vi "CreateLogStopNode.vi"(7 "DOM Document":refnum<k20>, 8 "Error In":errorcluster, 11 "Log Stop Configuration":T1={"Trigger Type"=enum."User", "Timer (sec)"=0.0, "File Size (MB)"=256, "Digital IO Line"=1, "Digital IO Edge"=enum."Rising"}) -> (0 "Error Out":errorcluster, 3 "Stop Node":refnum<k20>)   [LabVIEW 2013]
uses:
  LogStopConfiguration.ctl
  LogStopTriggerType.ctl
  LogDigitalIOTriggerEdge.ctl
  libs/LV-Utilities/LV-Utilities.lvlib
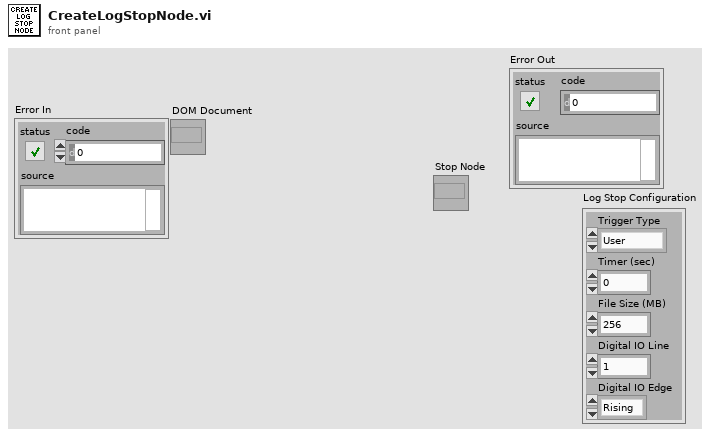
[diagram p1: front panel]
types:
  T1 = typedef "LogStopConfiguration.ctl" = cluster{"Trigger Type":T2, "Timer (sec)":dbl, "File Size (MB)":u32, "Digital IO Line":u8, "Digital IO Edge":T3}
  T2 = typedef "LogStopTriggerType.ctl" = enum16{"None", "User", "Timer", "File Size", "Digital IO"}
  T3 = typedef "LogDigitalIOTriggerEdge.ctl" = enum16{"Rising", "Falling"}
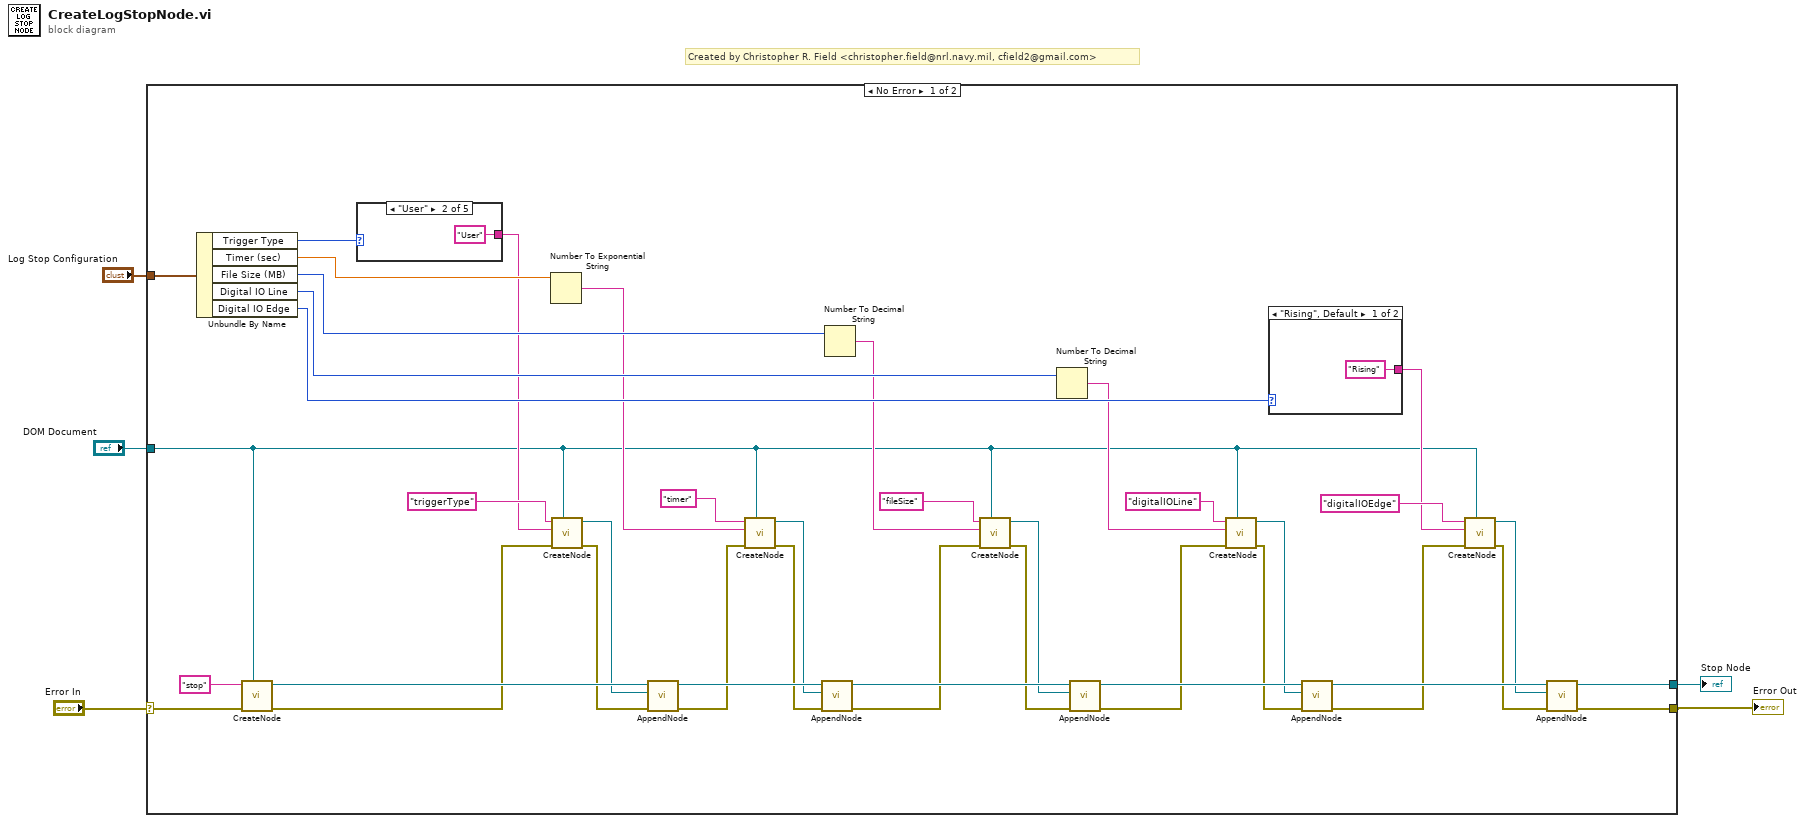
[diagram p0: block diagram]
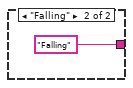
[diagram p2: hidden frame]
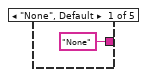
[diagram p3: hidden frame]
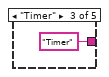
[diagram p4: hidden frame]
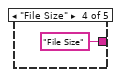
[diagram p5: hidden frame]
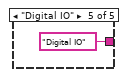
[diagram p6: hidden frame]
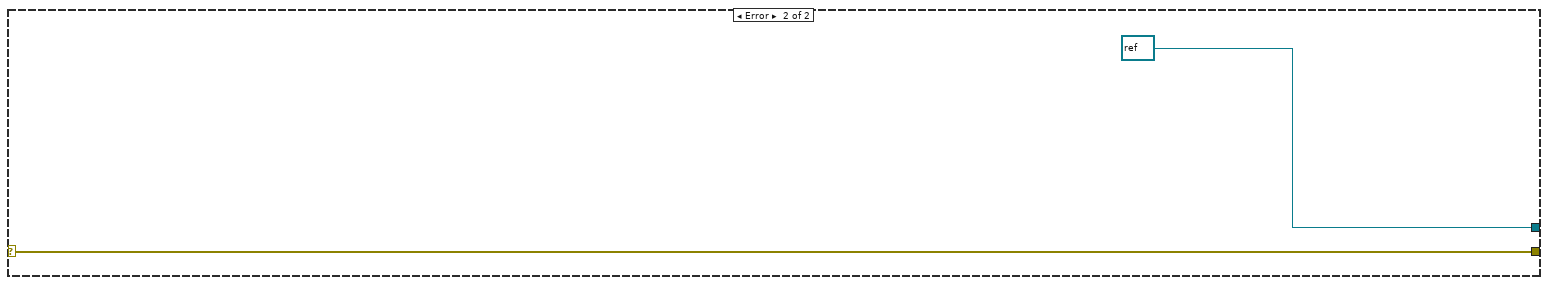
[diagram p7: hidden frame]
diagram:
  # "Created by Christopher R. Field <christopher.field@nrl.navy.mil, cfield2@gmail.com>"
  n1 = case shown="No Error" "Error In" {
    selector: "Error In" -> [w30 w55]
    tunnel: "DOM Document" -> [w19 _]
    tunnel: [w23 refnum<k20> refnum ("Wirings Node 2")] -> w3
    tunnel: [w22 w55] -> w2
    tunnel: "Log Stop Configuration" -> [w46 _]
    frame No Error {
      n2 = Unbundle By Name(w46) -> ("Trigger Type"=w45:T2, "Timer (sec)"=w44:dbl, "File Size (MB)"=w43:u32, "Digital IO Line"=w41:u8, "Digital IO Edge"=w42:T3)
      n3 = call "CreateNode.vi"("DOM Document"=w19, "Error In"=w30, "Tag Name"="stop") -> ("Error out"=w6:errorcluster, "Node"=w28:refnum<k20>)  [unwired: 7 in]
      n4 = case shown="\"User\"" w45 {
        tunnel: ["None" "User" "Timer" "File Size" "Digital IO"] -> w39
        frame "None", Default {
        }
        frame "User" {
        }
        frame "Timer" {
        }
        frame "File Size" {
        }
        frame "Digital IO" {
        }
      }
      n5 = Number To Exponential String(number=w44) -> (E-format string=w31:string)  [unwired: 3 in]
      n6 = call "CreateNode.vi"("DOM Document"=w19, "Error In"=w6, "Text"=w39, "Tag Name"="triggerType") -> ("Error out"=w8:errorcluster, "Node"=w7:refnum<k20>)  [unwired: 6 in]
      n7 = call "AppendNode.vi"("Error In"=w8, "Child Node"=w7, "Parent Node In"=w28) -> ("Error Out"=w9:errorcluster, "Parent Node Out"=w27:refnum<k20>)  [unwired: 7 in]
      n8 = call "CreateNode.vi"("DOM Document"=w19, "Error In"=w9, "Text"=w31, "Tag Name"="timer") -> ("Error out"=w11:errorcluster, "Node"=w10:refnum<k20>)  [unwired: 6 in]
      n9 = call "AppendNode.vi"("Error In"=w11, "Child Node"=w10, "Parent Node In"=w27) -> ("Error Out"=w12:errorcluster, "Parent Node Out"=w26:refnum<k20>)  [unwired: 7 in]
      n10 = Number To Decimal String(number=w43) -> (decimal integer string=w32:string)  [unwired: 1 in]
      n11 = call "CreateNode.vi"("DOM Document"=w19, "Error In"=w12, "Text"=w32, "Tag Name"="fileSize" ("Text")) -> ("Error out"=w14:errorcluster, "Node"=w13:refnum<k20>)  [unwired: 6 in]
      n12 = Number To Decimal String(number=w41) -> (decimal integer string=w33:string)  [unwired: 1 in]
      n13 = call "AppendNode.vi"("Error In"=w14, "Child Node"=w13, "Parent Node In"=w26) -> ("Error Out"=w15:errorcluster, "Parent Node Out"=w25:refnum<k20>)  [unwired: 7 in]
      n14 = call "CreateNode.vi"("DOM Document"=w19, "Error In"=w15, "Text"=w33, "Tag Name"="digitalIOLine") -> ("Error out"=w17:errorcluster, "Node"=w16:refnum<k20>)  [unwired: 6 in]
      n15 = case shown="\"Rising\", Default" w42 {
        tunnel: ["Rising" "Falling"] -> w34
        frame "Rising", Default {
        }
        frame "Falling" {
        }
      }
      n16 = call "AppendNode.vi"("Error In"=w17, "Child Node"=w16, "Parent Node In"=w25) -> ("Error Out"=w18:errorcluster, "Parent Node Out"=w24:refnum<k20>)  [unwired: 7 in]
      n17 = call "CreateNode.vi"("DOM Document"=w19, "Error In"=w18, "Text"=w34, "Tag Name"="digitalIOEdge") -> ("Error out"=w21:errorcluster, "Node"=w20:refnum<k20>)  [unwired: 6 in]
      n18 = call "AppendNode.vi"("Error In"=w21, "Child Node"=w20, "Parent Node In"=w24) -> ("Error Out"=w22:errorcluster, "Parent Node Out"=w23:refnum<k20>)  [unwired: 7 in]
    }
    frame Error {
    }
  }
  "Stop Node" <- w3
  "Error Out" <- w2
